vi "incrementNofThreads.vi"(0 "HGF_ThreadPool":refnum<class "HGF_ThreadPool.lvclass">, 2 "threadRef":refnum<vi>, 3 "stopOccurrence":refnum<k4>, 5 "error in (no error)":errorcluster) -> (14 "dup HGF_ThreadPool":refnum<class "HGF_ThreadPool.lvclass">, 19 "error out":errorcluster)   [LabVIEW 2014, in "HGF_BaseClasses.lvlib" / "HGF_ThreadPool.lvclass"]
doc: "Increment number of active threads and append thread reference.\n\n<b>Attention:</b> This VI should be call from HGF_ThreadWorker.startThread.vi only!"
uses:
  HGF_ThreadPool.lvclass
  HGF_Auxiliary/HGF_Auxiliary.lvlib
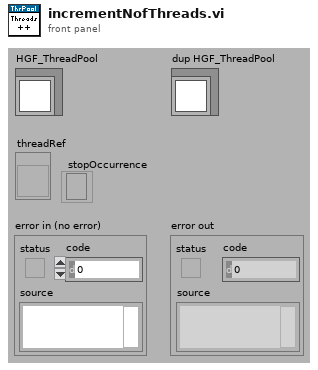
[diagram p1: front panel]
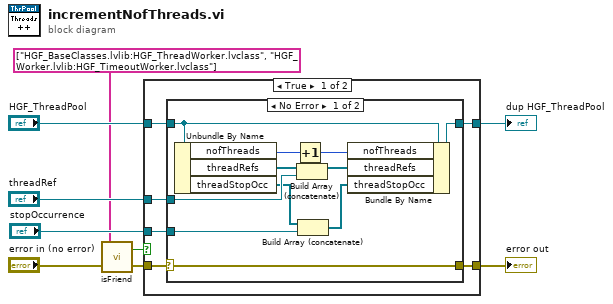
[diagram p0: block diagram]
diagram:
  n1 = call "isFriend.vi"("error in (no error)"="error in (no error)", "Friends"=string[] ["HGF_BaseClasses.lvlib:HGF_ThreadWorker.lvclass", "HGF_Worker.lvlib:HGF_TimeoutWorker.lvclass"]) -> ("error out"=w3:errorcluster, "isFriend?"=w1:bool)
  n2 = case shown="True" w1 {
    tunnel: w3 -> [w15 w29]
    tunnel: [w14 w29] -> w9
    tunnel: "HGF_ThreadPool" -> [w13 w30]
    tunnel: [w12 w30] -> w7
    tunnel: "threadRef" -> [w11 _]
    tunnel: "stopOccurrence" -> [w10 _]
    frame True {
      n3 = case shown="No Error" w15 {
        selector: w15 -> [w26 w27]
        tunnel: [w26 w27] -> w14
        tunnel: [w24 w28] -> w12
        tunnel: w13 -> [w25 w28]
        tunnel: w11 -> [w20 _]
        tunnel: w10 -> [w17 _]
        frame No Error {
          n4 = Unbundle By Name(w25) -> ("nofThreads"=w23:i32, "threadRefs"=w21:refnum<vi>[], "threadStopOcc"=w18:refnum<k4>[])
          n5 = Increment(x=w23) -> (x+1=w22:i32)
          n6 = Build Array (concatenate)(w21, w20) -> (w19:refnum<vi>[])
          n7 = Build Array (concatenate)(w18, w17) -> (w16:refnum<k4>[])
          n8 = Bundle By Name(cluster=w25, "nofThreads"=w22, "threadRefs"=w19, "threadStopOcc"=w16) -> (w24:refnum<class "HGF_ThreadPool.lvclass">)
        }
        frame Error {
        }
      }
    }
    frame False {
    }
  }
  "error out" <- w9
  "dup HGF_ThreadPool" <- w7
